vi "rx FM.vi"() -> ()   [LabVIEW 2012]
uses:
  <instrlib>/niUSRP/niUSRP Fetch Rx Data (CDB Cluster).vi
  <vilib>/addons/Modulation/niAMT.lvlib
panel:
  out "FM demodulated waveform":waveform(dbl)(graph)={"t0"=timestamp(17645.74410987 s since 1904-01-01), "dt"=5e-06, "Y"=[]}
  in  "carrier frequency":dbl=434000000.0 format="%#_6p"
  in  "Rx IQ rate":dbl=200000.0
  out "IQ Graph":cluster{dbl[], dbl[]}(graph)
  in  "number of samples":i64=20480
  in  "Stop":bool
  out "Waveform Graph":dbl[][](graph)
  out "error out":errorcluster
  out "coerced gain":dbl=30.0 format="%#_6f"
  out "coerced carrier frequency":dbl=434000000.0092859 format="%#_6p"
  out "coerced IQ rate":dbl=200000.0 format="%.6p"
  in  "active antenna":string="RX2"
  in  "rx gain":dbl=30.0 format="%#_6f"
  in  "device names":refnum<k15>="10.100.1.125"
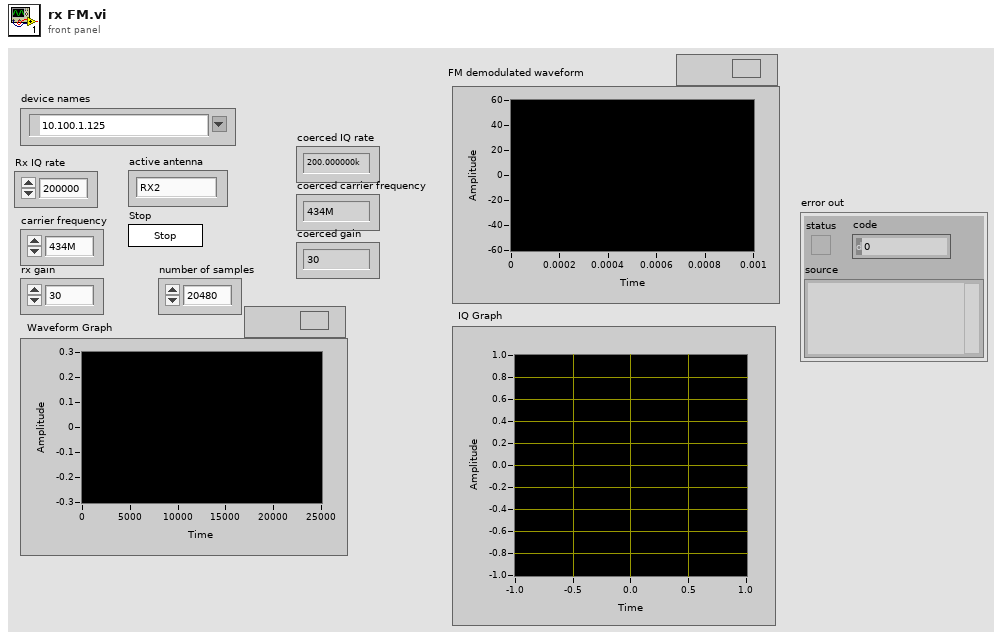
[diagram p1: front panel]
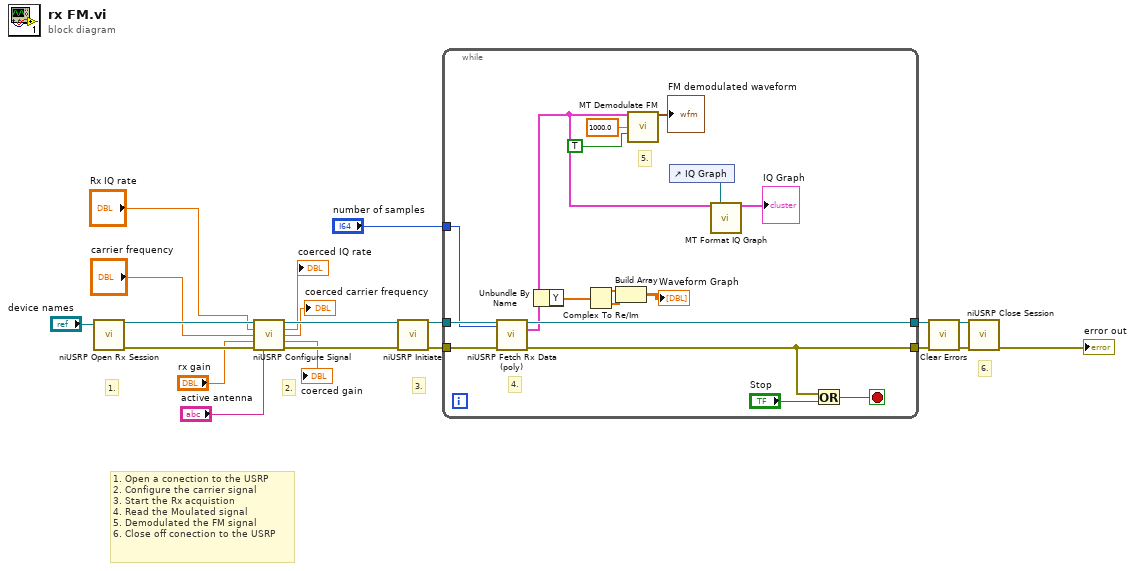
[diagram p0: block diagram]
diagram:
  # "1. Open a conection to the USRP\n2. Configure the carrier signal\n3. Start the Rx acquistion\n4. Read the Moulated signal\n5. Demodulated the FM signal\n6. Close off conection to the USRP"
  # "6."
  # "3."
  # "2."
  # "1."
  n1 = call <instrlib>:"niUSRP Open Rx Session.vi"("device names"="device names") -> ("session handle out"=w18:refnum<k15>, "error out"=w17:errorcluster)  [unwired: 13 in]
  n2 = call <instrlib>:"niUSRP Configure Signal.vi"("session handle"=w18, "IQ rate"="Rx IQ rate", "carrier frequency"="carrier frequency", "gain"="rx gain", "error in (no error)"=w17, "active antenna"="active antenna") -> ("session handle out"=w13:refnum<k15>, "coerced IQ rate"=→"coerced IQ rate":dbl, "coerced carrier frequency"=→"coerced carrier frequency":dbl, "coerced gain"=→"coerced gain":dbl, "error out"=w14:errorcluster)  [unwired: 5 in]
  n3 = call <instrlib>:"niUSRP Initiate.vi"("session handle"=w13, "error in (no error)"=w14) -> ("session handle out"=w6:refnum<k15>, "error out"=w5:errorcluster)  [unwired: 12 in]
  n4 = while {
    tunnel: w6 -> [w36]
    tunnel: w5 -> [w35]
    tunnel: [w34] -> w4
    tunnel: [w26] -> w3
    tunnel: "number of samples" -> [w20]
    stop <- w30 stop-if-true
    # "5."
    # "4."
    n5 = call-poly <instrlib>:"niUSRP Fetch Rx Data (poly).vi"("session handle"=w36, "number of samples"=w20, "error in (no error)"=w35) -> ("session handle out"=w34:refnum<k15>, "data"=w27:cluster{"t0":dbl, "dt":dbl, "Y":cdb[]}, "error out"=w26:errorcluster)  [unwired: 9 in, 1 out]
    n6 = Unbundle By Name(w27) -> ("Y"=w28:cdb[])
    n7 = Complex To Re/Im(x + iy=w28) -> (x=w31:dbl[], y=w33:dbl[])
    n8 = Build Array(w31, w33) -> (→"Waveform Graph":dbl[][])
    n9 = call <vilib>:"MT Demodulate FM.vi"("FM modulated waveform"=w27, "FM deviation (Hz)"=1000.0, "carrier correction? (F)"=TRUE) -> ("FM demodulated waveform"=→"FM demodulated waveform":waveform(dbl))  [unwired: 10 in, 2 out]
    n10 = control-ref of="IQ Graph"() -> (w21:refnum<vi>)
    n11 = call <vilib>:"MT Format IQ Graph.vi"("IQ data (complex) in"=w27, "IQ graph reference"=w21) -> ("IQ Graph"=→"IQ Graph":cluster{dbl[], dbl[]})  [unwired: 2 in, 11 out]
    n12 = Or(x=w26, y="Stop") -> (x .or. y?=w30:bool)
  }
  n13 = call <vilib>:"Clear Errors.vi"("error in (no error)"=w3) -> ("error out"=w1:errorcluster)  [unwired: 6 in]
  n14 = call <instrlib>:"niUSRP Close Session.vi"("session handle"=w4, "error in (no error)"=w1) -> ("error out"=→"error out":errorcluster)  [unwired: 13 in]
